vi "Read debugLevel.vi"(8 "error in (no error)":errorcluster, 11 "MccDebug in":refnum<class "MccDebug.lvclass">) -> (0 "error out":errorcluster, 2 "debugLevel":T1, 3 "MccDebug out":refnum<class "MccDebug.lvclass">)   [LabVIEW 2022 SP3, in "TCSDataDefinitions.lvlib" / "TCSMountControlCommand.lvlib" / "CommandsForAllAxes.lvlib" / "MccDebug.lvclass"]
uses:
  MccDebug.lvclass
  TCSCommand/Enumerations/TCSDebuLevelTypes.ctl
  MccDebug.lvclass/MccDebug.ctl
  TCSCommand/TCSCommand.lvlib
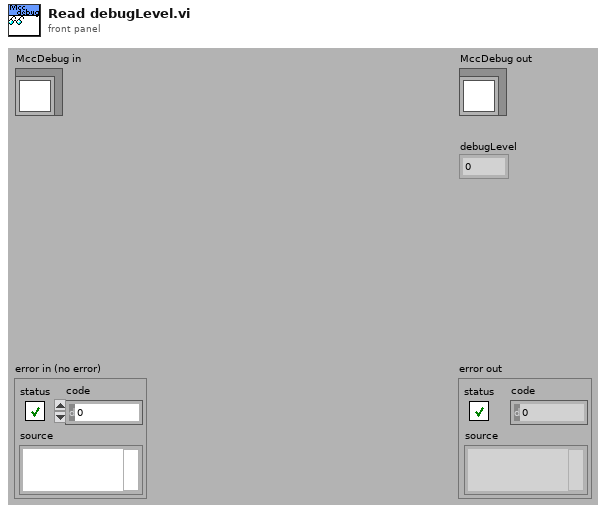
[diagram p1: front panel]
types:
  T1 = typedef "TCSDataDefinitions.lvlib/TCSCommand.lvlib/TCSDebuLevelTypes.ctl" = enum16{"0", "1", "2", "3", "4", "5", "6", "7", "8", "9", "10"}
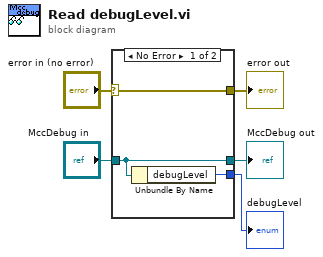
[diagram p0: block diagram]
diagram:
  n1 = case shown="No Error" "error in (no error)" {
    selector: "error in (no error)" -> [w8 w9]
    tunnel: [w8 w9] -> w4
    tunnel: [w7 w10] -> w2
    tunnel: "MccDebug in" -> [w7 w10]
    tunnel: [w6 _] -> w1
    frame No Error {
      n2 = Unbundle By Name(w7) -> ("debugLevel"=w6:T1)
    }
    frame Error {
    }
  }
  "error out" <- w4
  "MccDebug out" <- w2
  "debugLevel" <- w1
